vi "SerialWrite.vi"(8 "error in (no error)":errorcluster caption="错误输入（无错误）", 10 "串口写入":string, 11 "serial 输入":refnum<class "serial.lvclass">) -> (0 "error out":errorcluster caption="错误输出", 2 "返回数":u32, 3 "serial 输出":refnum<class "serial.lvclass">)   [LabVIEW 2019, in "serial.lvclass"]
uses:
  serial.lvclass
  serial.lvclass/serial.ctl
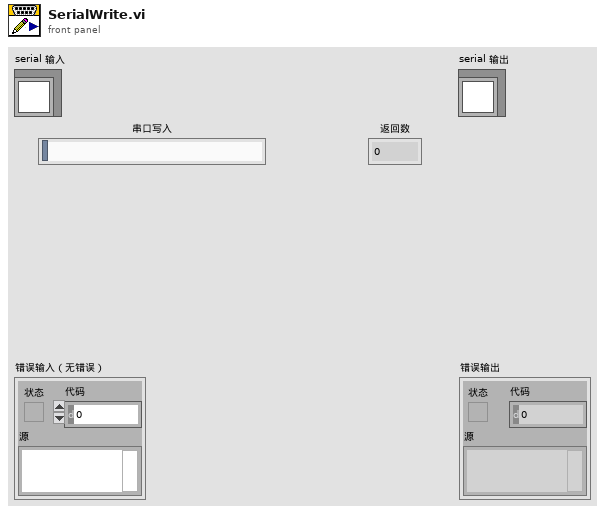
[diagram p1: front panel]
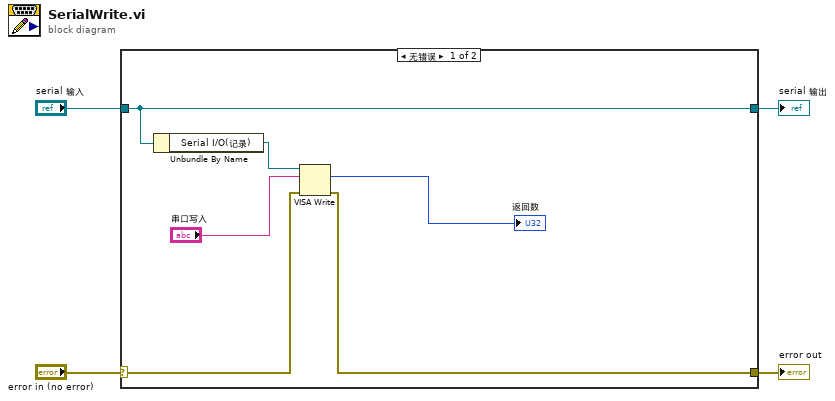
[diagram p0: block diagram]
diagram:
  n1 = case shown="无错误" "error in (no error)" {
    selector: "error in (no error)" -> [w6 w12]
    tunnel: [w5 w12] -> w3
    tunnel: [w10 w11] -> w1
    tunnel: "serial 输入" -> [w10 w11]
    frame No Error {
      n2 = Unbundle By Name(w10) -> ("Serial I/O(记录)"=w9:refnum<visa-resource-name>)
      n3 = VISA Write(VISA resource name=w9, write buffer="串口写入", error in (no error)=w6) -> (return count=→"返回数":u32, error out=w5:errorcluster)  [unwired: 1 out]
    }
    frame Error {
    }
  }
  "error out" <- w3
  "serial 输出" <- w1
